vi "SQLite Get Foreign Key List.vi"(8 "error in":errorcluster, 10 "Table Name":string="test", 11 "SQLite Connection":refnum<class "Connection.lvclass">) -> (0 "error out":errorcluster, 2 "Foreign Key List":T1[](array[typedef]), 3 "Dup SQLite Connection":refnum<class "Connection.lvclass">)   [LabVIEW 2021, in "EDT SQLite+.lvlib"]
uses:
  EDT SQLite+.lvlib
  SQLite Foreign Key.ctl
  SQLite Reaction Type.ctl
  <vilib>/drjdpowell/SQLite Library/SQL Connection/Connection.lvclass
  <vilib>/drjdpowell/SQLite Library/SQL Statement/SQL Statement.lvclass/SQL Statement.ctl
  <vilib>/drjdpowell/SQLite Library/SQL Statement/Column I64.vi
  <vilib>/drjdpowell/SQLite Library/SQL Statement/Error Message.vi
  <vilib>/drjdpowell/SQLite Library/SQL Statement/Column String.vi
  <vilib>/drjdpowell/SQLite Library/SQL Statement/SQL Statement.lvclass
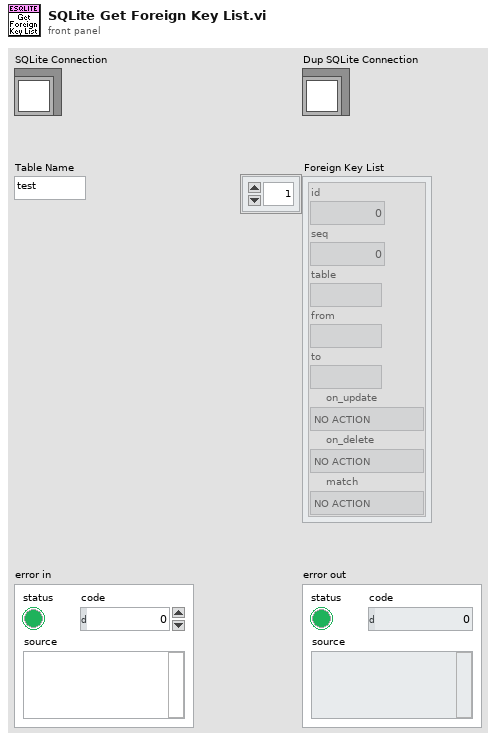
[diagram p1: front panel]
types:
  T1 = typedef "EDT SQLite+.lvlib/SQLite Foreign Key.ctl" = cluster{"id":i64, "seq":i64, "table":string, "from":string, "to":string, "on_update":T2, "on_delete":T2, "match":T2}
  T2 = typedef "EDT SQLite+.lvlib/SQLite Reaction Type.ctl" = enum16{"NO ACTION", "SET NULL", "SET DEFAULT", "CASCADE", "RESTRICT", "NONE"}
  T3 = cluster{"Column:Get Column I64":i64, "Column:Get Column I64":i64, "Column:Get Column String":string, "Column:Get Column String":string, "Column:Get Column String":string, "SQLite Reaction Type":T2, "SQLite Reaction Type":T2, "SQLite Reaction Type":T2}
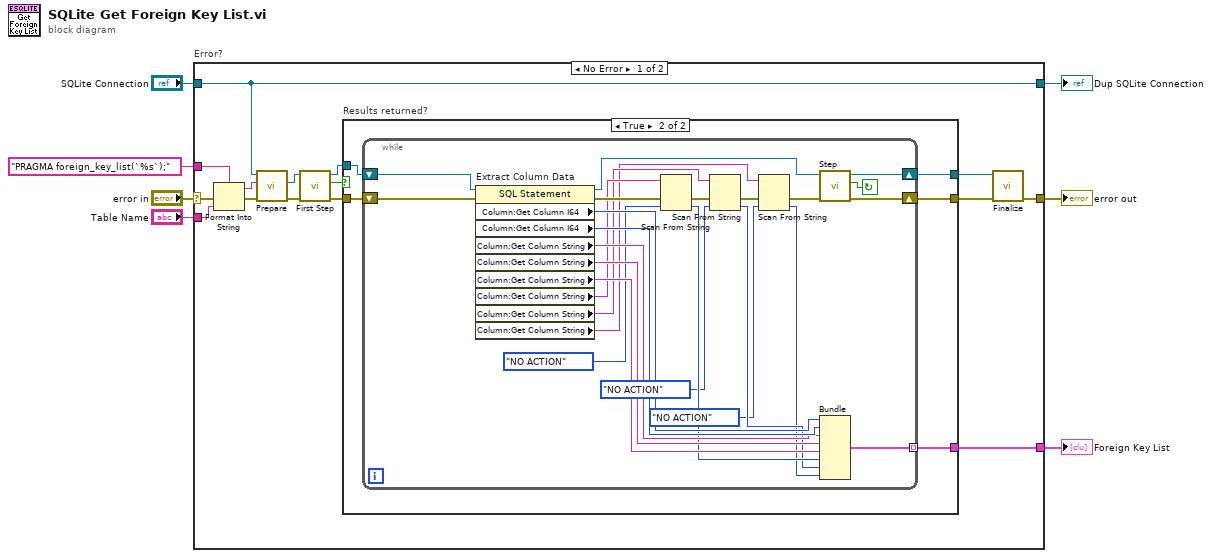
[diagram p0: block diagram]
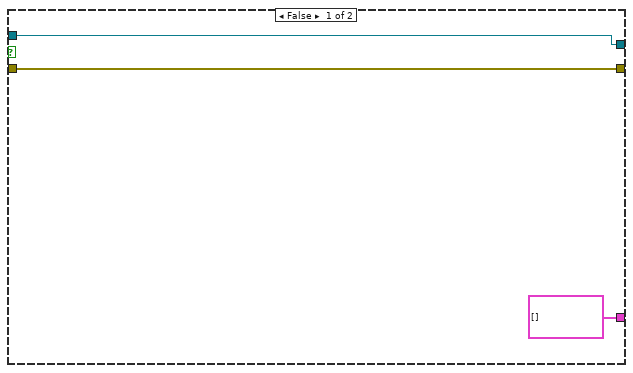
[diagram p2: hidden frame]
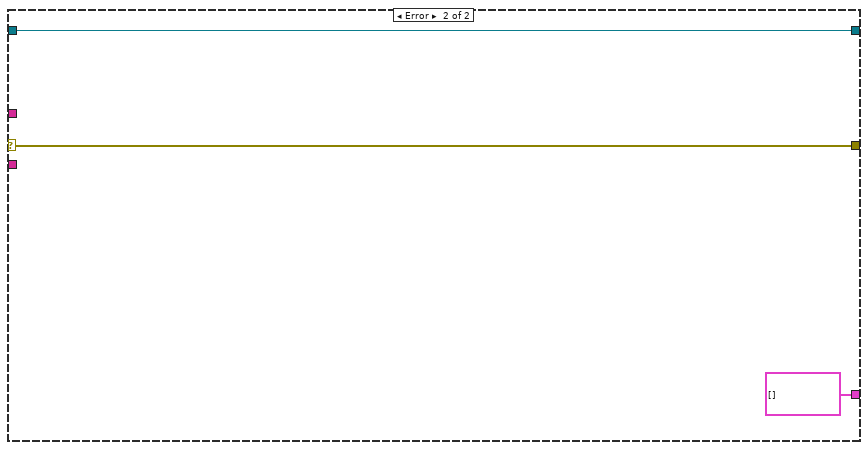
[diagram p3: hidden frame]
diagram:
  n1 = case "Error?" shown="No Error" "error in" {
    selector: "error in" -> [w22 w58]
    tunnel: "Table Name" -> [w21 _]
    tunnel: [w19 w58] -> w5
    tunnel: "SQLite Connection" -> [w20 w57]
    tunnel: [w20 w57] -> w3
    tunnel: [w18 T1[] [] ("Foreign Key List")] -> w2
    tunnel: "PRAGMA foreign_key_list(`%s`);" ("SELECT  statement") -> [w8 _]
    frame No Error {
      n2 = Format Into String(format string=w8, error in=w22, w21) -> (resulting string=w17:string, error out=w9:errorcluster)  [unwired: 1 in]
      n3 = call <vilib>:"Prepare.vi"("error in (no error)"=w9, "SQL"=w17, "SQLite Connection in"=w20) -> ("error out"=w10:errorcluster, "SQL Statement"=w11:refnum<class "SQL Statement.lvclass">)  [unwired: 4 in, 3 out]
      n4 = call <vilib>:"First Step.vi"("error in (no error)"=w10, "SQL Statement in"=w11) -> ("error out"=w13:errorcluster, "Row returned"=w12:bool, "SQL Statement"=w14:refnum<class "SQL Statement.lvclass">)  [unwired: 7 in]
      n5 = case "Results returned?" shown="True" w12 {
        tunnel: [w25 w30] -> w15
        tunnel: [w24 w29] -> w16
        tunnel: w14 -> [w25 w28]
        tunnel: w13 -> [w24 w27]
        tunnel: [T1[] [] ("Foreign Key List") w26] -> w18
        frame False {
        }
        frame True {
          n6 = while "For each row..." {
            shift-right: [w55] -> w30
            shift-left: w28 -> [w53]
            shift-right: [w54] -> w29
            shift-left: w27 -> [w52]
            tunnel: [w44] -> w26 mode=indexing
            stop <- w51 continue-if-true
            n7 = property on="Extract Column Data" class="SQL Statement"(reference=w53, error in=w52) -> (reference out=w50:refnum<class "SQL Statement.lvclass">, error out=w43:errorcluster, "Column:Get Column I64"=w49:i64, "Column:Get Column I64"=w48:i64, "Column:Get Column String"=w47:string, "Column:Get Column String"=w46:string, "Column:Get Column String"=w45:string, "Column:Get Column String"=w42:string, "Column:Get Column String"=w37:string, "Column:Get Column String"=w32:string)
            n8 = Scan From String(input string=w42, error in=w43, default 1=SQLite_Reaction_Type."NO ACTION" ("SQLite Reaction Type")) -> (error out=w38:errorcluster, output 1=w40:T2)  [unwired: 2 in, 2 out]
            n9 = Scan From String(input string=w37, error in=w38, default 1=SQLite_Reaction_Type."NO ACTION" ("SQLite Reaction Type")) -> (error out=w34:errorcluster, output 1=w36:T2)  [unwired: 2 in, 2 out]
            n10 = Scan From String(input string=w32, error in=w34, default 1=SQLite_Reaction_Type."NO ACTION" ("SQLite Reaction Type")) -> (error out=w33:errorcluster, output 1=w31:T2)  [unwired: 2 in, 2 out]
            n11 = call <vilib>:"Step.vi"("error in (no error)"=w33, "SQL Statement in"=w50) -> ("error out"=w54:errorcluster, "Row returned"=w51:bool, "SQL Statement"=w55:refnum<class "SQL Statement.lvclass">)  [unwired: 7 in]
            n12 = Bundle("Column:Get Column I64"=w49, "Column:Get Column I64"=w48, "Column:Get Column String"=w47, "Column:Get Column String"=w46, "Column:Get Column String"=w45, "SQLite Reaction Type"=w40, "SQLite Reaction Type"=w36, "SQLite Reaction Type"=w31) -> (w44:T3)  [unwired: 1 in]
          }
        }
      }
      n13 = call <vilib>:"Finalize.vi"("error in (no error)"=w16, "SQL Statement in"=w15) -> ("error out"=w19:errorcluster)  [unwired: 9 in]
    }
    frame Error {
    }
  }
  "error out" <- w5
  "Foreign Key List" <- w2
  "Dup SQLite Connection" <- w3
